vi "GetAttributes.vi"(0 "ClassReaderNative in":refnum<class "ClassReaderNative.lvclass">, 1 "OnlyGetReference":bool, 5 "error in (no error)":errorcluster) -> (14 "ClassReaderNative out":refnum<class "ClassReaderNative.lvclass">, 15 "ObjectAttributes":T1[](array[typedef])=[{"name"="MyU8", "type"=enum."UINT8", "dimension"=0, "typeName"="", "typePath"=path "", "visibility"=enum."Protected"}, {"name"="MyStrArray", "type"=enum."STRING", "dimension"=1, "typeName"="", "typePath"=path "", "visibility"=enum."Protected"}], 16 "ClassAttributes":T1[](array[typedef])=[{"name"="MyU8", "type"=enum."UINT8", "dimension"=0, "typeName"="", "typePath"=path "", "visibility"=enum."Protected"}, {"name"="MyStrArray", "type"=enum."STRING", "dimension"=1, "typeName"="", "typePath"=path "", "visibility"=enum."Protected"}], 17 "ObjectAttributeReference":refnum<vi>, 18 "ClassAttributeReference":refnum<vi>, 19 "error out":errorcluster)   [LabVIEW 2012, in "ClassReaderNative.lvclass"]
uses:
  <resource>/Framework/Providers/Open_GDS/ClassProviders/Provider_LvNativeClass/ClassReaderNative_class/ClassReaderNative.lvclass
  <resource>/Framework/Providers/Open_GDS/UML/ReversedEngineering/ReversedEngineering AttributeInfoType.ctl
  <resource>/Framework/Providers/Open_GDS/ClassProviders/Common/CommonVIs/CommonVIs_AttributeDataType.ctl
  <resource>/Framework/Providers/Open_GDS/UML/UMLEditor/UMLEditor_VisibilityType.ctl
  <resource>/Framework/Providers/Open_GDS/ClassProviders/Provider_LvNativeClass/ClassReaderNative_class/ClassReaderNative.lvclass/ClassReaderNative.ctl
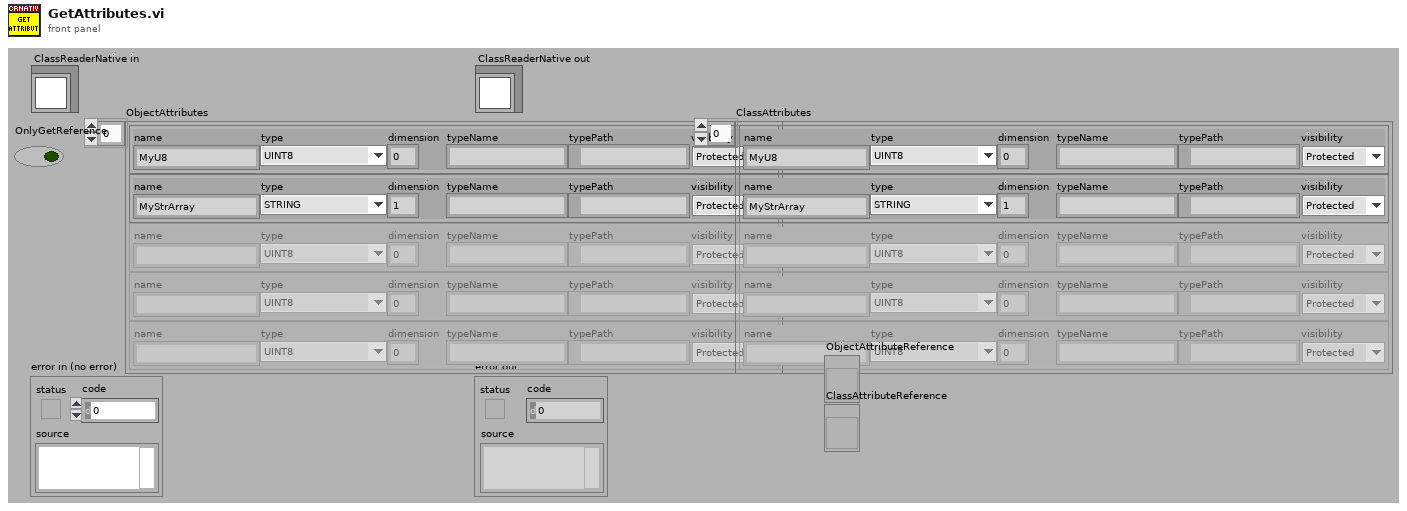
[diagram p1: front panel]
types:
  T1 = typedef "ReversedEngineering AttributeInfoType.ctl" = cluster{"name":string, "type":T2, "dimension":i32, "typeName":string, "typePath":path, "visibility":T3}
  T2 = typedef "CommonVIs_AttributeDataType.ctl" = enum16{"UINT8", "INT8", "UINT16", "INT16", "UINT32", "INT32", "UINT64", "INT64", "SGL", "DBL", "EXT", "CSG", "CDB", "CXT", "TimeStamp", "STRING", "PATH", "BOOL", "ENUM", "RefNum", "VIRefNum", "LabVIEW Class", "Cluster", "Variant", "TypeDef", "Waveform", "LabVIEW Object", "Other", "void"}
  T3 = typedef "UMLEditor_VisibilityType.ctl" = enum16{"Public", "Private", "Protected"}
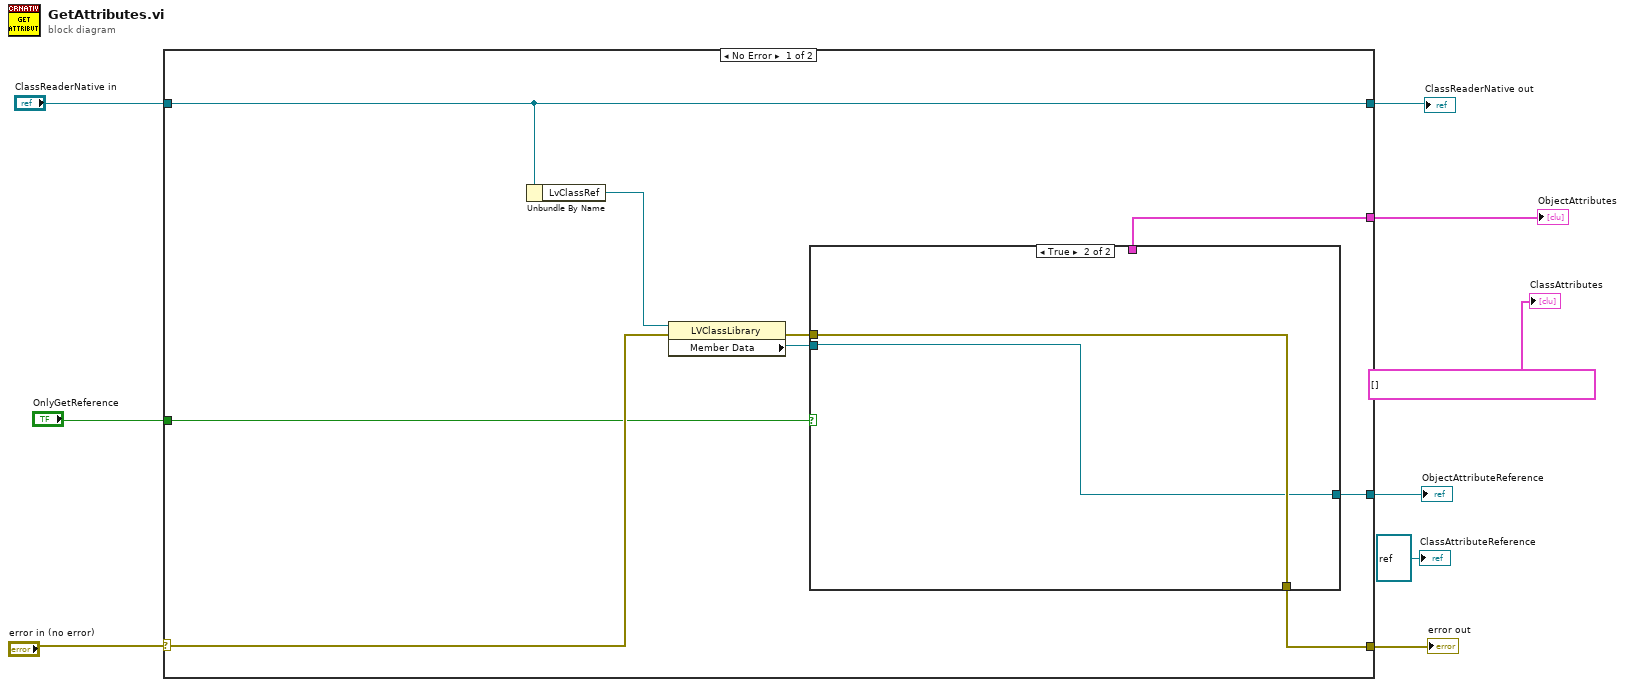
[diagram p0: block diagram]
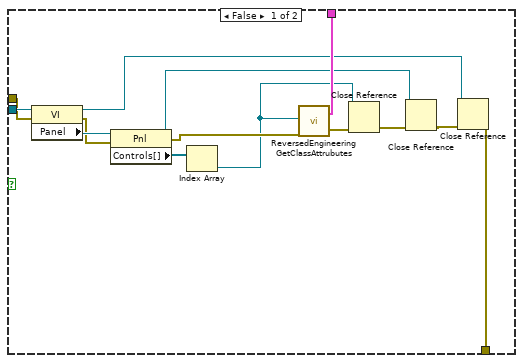
[diagram p2: hidden frame]
diagram:
  n1 = case shown="No Error" "error in (no error)" {
    selector: "error in (no error)" -> [w15 w35]
    tunnel: "ClassReaderNative in" -> [w14 w36]
    tunnel: [w14 w36] -> w7
    tunnel: [w12 w35] -> w6
    tunnel: [w16 _] -> w5
    tunnel: "OnlyGetReference" -> [w10 _]
    tunnel: [w11 _] -> w2
    frame No Error {
      n2 = Unbundle By Name(w14) -> ("LvClassRef"=w13:refnum<vi>)
      n3 = property class="LVClassLibrary"(reference=w13, error in=w15) -> (error out=w17:errorcluster, "Member Data"=w18:refnum<vi>)  [unwired: 1 out]
      n4 = case shown="True" w10 {
        tunnel: w18 -> [w32 w33]
        tunnel: w17 -> [w31 w34]
        tunnel: [w26 _] -> w16
        tunnel: [w19 w34] -> w12
        tunnel: [_ w33] -> w11
        frame False {
          n5 = property class="VI"(reference=w32, error in=w31) -> (reference out=w21:refnum<vi>, error out=w27:errorcluster, "Panel"=w29:refnum<vi>)
          n6 = property class="Pnl"(reference=w29, error in=w27) -> (reference out=w23:refnum<vi>, error out=w28:errorcluster, "Controls[]"=w30:refnum<vi>[])
          n7 = Index Array(array=w30) -> (element=w25:refnum<vi>)  [unwired: 1 in]
          n8 = call <resource>:"ReversedEngineering GetClassAttrubutes.vi"("CtlRefnum"=w25, "error in (no error)"=w28) -> ("attributeInfo"=w26:T1[], "error out"=w20:errorcluster)  [unwired: 15 in, 1 out]
          n9 = Close Reference(reference=w25, error in (no error)=w20) -> (error out=w24:errorcluster)
          n10 = Close Reference(reference=w23, error in (no error)=w24) -> (error out=w22:errorcluster)
          n11 = Close Reference(reference=w21, error in (no error)=w22) -> (error out=w19:errorcluster)
        }
        frame True {
        }
      }
    }
    frame Error {
    }
  }
  "ClassReaderNative out" <- w7
  "error out" <- w6
  "ObjectAttributes" <- w5
  "ObjectAttributeReference" <- w2
  "ClassAttributes" <- T1[] [] ("ClassAttributes")
  "ClassAttributeReference" <- refnum<vi> refnum ("ClassAttributeReference")
